vi "Open_gas_valve.vi"(11 "error in":errorcluster) -> (3 "error out":errorcluster)   [LabVIEW 2017, in "Steps.lvlib"]
uses:
  Steps.lvlib
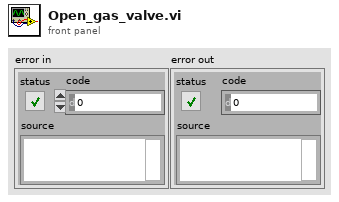
[diagram p1: front panel]
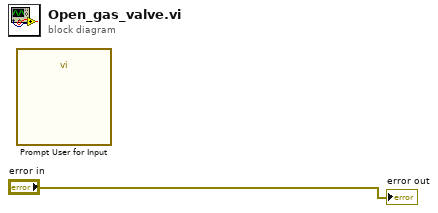
[diagram p0: block diagram]
diagram:
  n1 = call "Prompt User for Input"() -> ()  [unwired: 18 in, 2 out]
  "error out" <- "error in"
